vi "Update Message Capabilities.vi"(8 "error in (no error)":errorcluster, 11 "NodeDiscovery in":refnum<class "DiscoveryService.lvclass">) -> (0 "error out":errorcluster, 3 "NodeDiscovery out":refnum<class "DiscoveryService.lvclass">)   [LabVIEW 2020, in "Vecto.lvlib" / "DiscoveryService.lvclass"]
uses:
  DiscoveryService.lvclass
  DiscoveryService.lvclass/DiscoveryService.ctl
  proto/Discovery/Class/Msg.lvclass/Msg.ctl
  proto/Discovery/Class/Msg.lvclass
  Node Config/Node Config.lvclass
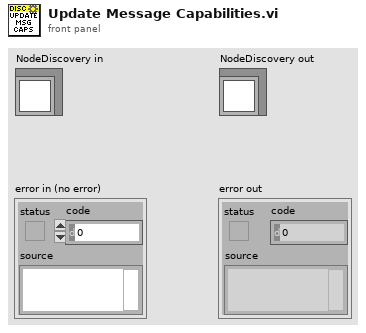
[diagram p1: front panel]
types:
  T1 = typedef "Discovery.lvlib/Data.ctl" = cluster{"node_id":u32, "name":string, "ip":u32, "status":string, "services":T2[], "capabilities":string[], "system":string, "cluster":string, "app_version":string, "cfg_version":string}
  T2 = typedef "Service.lvlib/Data.ctl" = cluster{"type":T3, "port":i32}
  T3 = typedef "ServiceType.lvlib/Enumeration.ctl" = enum16{"SERVICETYPE_UNKNOWN", "SERVICETYPE_TCPSERVER", "SERVICETYPE_HTTPSERVER"}
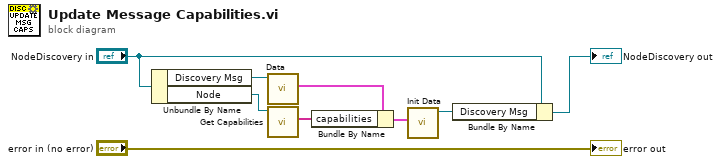
[diagram p0: block diagram]
diagram:
  n1 = Unbundle By Name("NodeDiscovery in") -> ("Discovery Msg"=w8:refnum<class "Msg.lvclass">, "Node"=w7:refnum<class "Node Config.lvclass">)
  n2 = call "Data.vi"("PB Msg Template in"=w8) -> ("Data"=w6:T1)  [unwired: 8 in, 2 out]
  n3 = call "Get Capabilities.vi"("Node Config in"=w7) -> ("Capabilities"=w5:string[])  [unwired: 8 in, 2 out]
  n4 = Bundle By Name(cluster=w6, "capabilities"=w5) -> (w4:T1)
  n5 = call "Init Data.vi"("Data"=w4) -> ("Msg out"=w3:refnum<class "Msg.lvclass">)  [unwired: 10 in]
  n6 = Bundle By Name(cluster="NodeDiscovery in", "Discovery Msg"=w3) -> (→"NodeDiscovery out":refnum<class "DiscoveryService.lvclass">)
  "error out" <- "error in (no error)"
